vi "Point Probe.vi"(1 "Point.lvclass":refnum<class "Point.lvclass">) -> (0 "Pause VI?":bool)   [LabVIEW 2017, in "Point.lvclass"]
doc: "This VI is a custom prove for the Point class."
uses:
  Point.lvclass
  Point.lvclass/Point.ctl
panel:
  out "Y":i16
  out "X":i16
  # "Point coordinates"
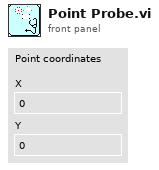
[diagram p1: front panel]
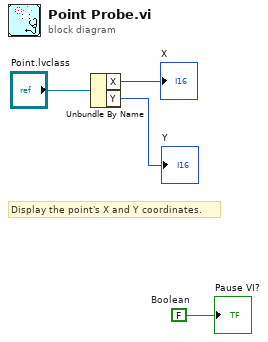
[diagram p0: block diagram]
diagram:
  w2 = FALSE  # Boolean
  # "Display the point's X and Y coordinates."
  n1 = Unbundle By Name("Point.lvclass") -> ("X"=→"X":i16, "Y"=→"Y":i16)
  "Pause VI?" <- w2
